vi "Write Triggers.vi"(8 "error in (no error)":errorcluster, 10 "Triggers":T1, 11 "FgenPluginsBase in":refnum<class "FgenPluginsBase.lvclass">) -> (0 "error out":errorcluster, 3 "FgenPluginsBase out":refnum<class "FgenPluginsBase.lvclass">)   [LabVIEW 2014, in "FgenPlugins.lvlib" / "FgenPluginsBase.lvclass"]
uses:
  FgenPluginsBase.lvclass
  TypeDefs/clTriggers.ctl
  TypeDefs/Trigger.ctl
  TypeDefs/TriggerType.ctl
  FgenPluginsBase.lvclass/FgenPluginsBase.ctl
  FgenPlugins.lvlib
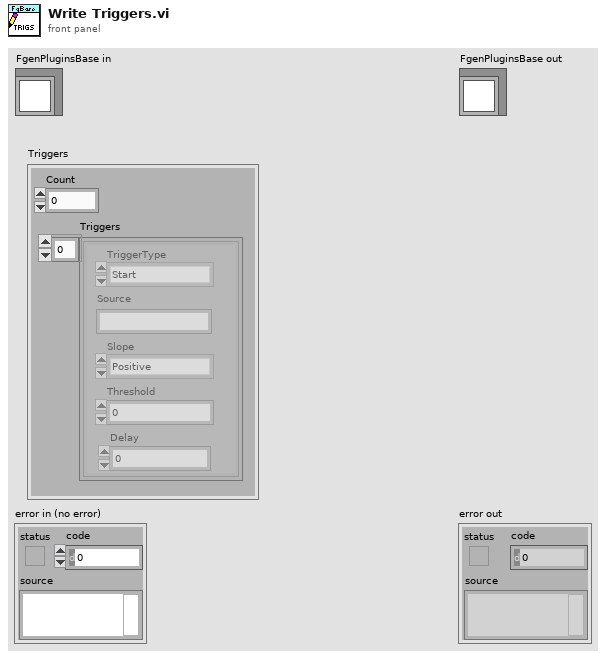
[diagram p1: front panel]
types:
  T1 = typedef "FgenPlugins.lvlib/clTriggers.ctl" = cluster{"Count":i32, "Triggers":T2[]}
  T2 = typedef "FgenPlugins.lvlib/Trigger.ctl" = cluster{"Source":string, "Slope":enum16{"Positive", "Negative", "Either"}, "Threshold":dbl, "Delay":dbl, "TriggerType":T3}
  T3 = typedef "FgenPlugins.lvlib/TriggerType.ctl" = enum16{"None", "Start", "Stop", "Hold", "Resume", "Advance"}
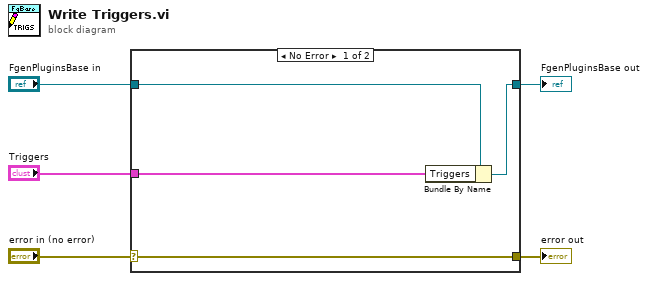
[diagram p0: block diagram]
diagram:
  n1 = case shown="No Error" "error in (no error)" {
    selector: "error in (no error)" -> [w9 w10]
    tunnel: [w9 w10] -> w4
    tunnel: [w7 w11] -> w2
    tunnel: "FgenPluginsBase in" -> [w8 w11]
    tunnel: "Triggers" -> [w6 _]
    frame No Error {
      n2 = Bundle By Name(cluster=w8, "Triggers"=w6) -> (w7:refnum<class "FgenPluginsBase.lvclass">)
    }
    frame Error {
    }
  }
  "error out" <- w4
  "FgenPluginsBase out" <- w2
